vi "Connect.vi"(6 "Priority (F)":bool, 8 "error in (no error)":errorcluster, 11 "Data":variant) -> (0 "error out":errorcluster)   [LabVIEW 2020, in "Wait.lvlib"]
uses:
  Wait.lvlib
  Private Controls/Module Action.ctl
  Private Controls/Element.ctl
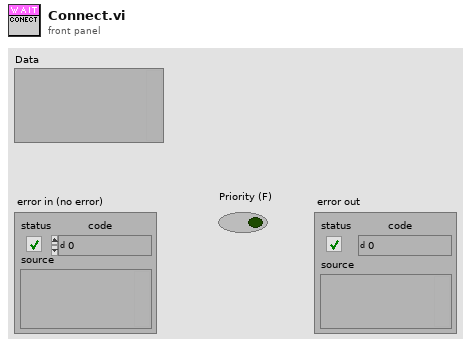
[diagram p1: front panel]
types:
  T1 = typedef "Wait.lvlib/Module Action.ctl" = enum16{"Initialise Module", "Start", "Wait", "Abort", "Error", "Exit"}
  T2 = typedef "Wait.lvlib/Element.ctl" = cluster{"Action":T3, "Data":variant}
  T3 = typedef "Wait.lvlib/Module Action.ctl" = enum16{"Initialise Module", "Connect", "Setup", "Pause", "Start", "Stop", "Wait: Time Elapsed", "Error", "Exit"}
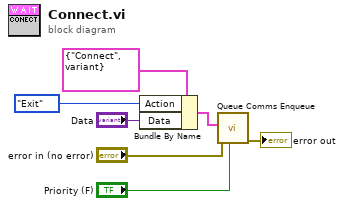
[diagram p0: block diagram]
diagram:
  n1 = Bundle By Name(cluster=T2 {"Action"=enum."Connect", "Data"=variant} ("Element"), "Action"=Module_Action."Exit", "Data"="Data") -> (w1:T2)
  n2 = call "Queue Comms Enqueue.vi"("Priority (F)"="Priority (F)", "error in (no error)"="error in (no error)", "Element"=w1) -> ("error out"=→"error out":errorcluster)  [unwired: 8 in]
